vi "WraparoundUpdate.vi"(9 "Data":i32[](array[numeric]), 10 "Location":u32, 11 "Accumulator":i32[](array[numeric])) -> (2 "NewLocation":u32, 3 "Accumulated":i32[](array[numeric]))   [LabVIEW 2014]
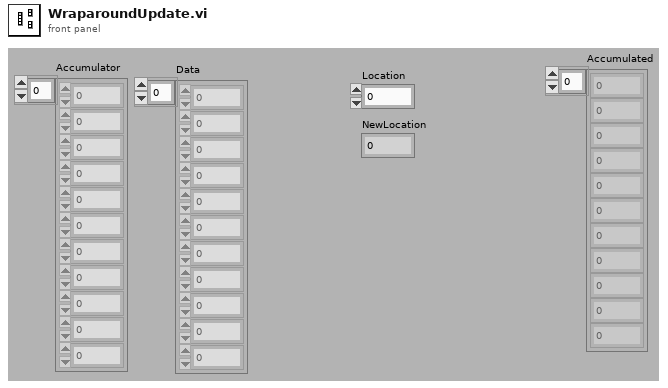
[diagram p1: front panel]
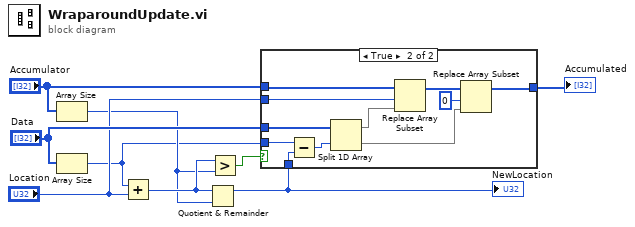
[diagram p0: block diagram]
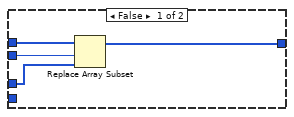
[diagram p2: hidden frame]
diagram:
  n1 = Array Size(array="Accumulator") -> (size(s)=w4:i32)
  n2 = Array Size(array="Data") -> (size(s)=w2:i32)
  n3 = Add(x=w2, y="Location") -> (x+y=w5:u32)
  n4 = Quotient & Remainder(x=w5, y=w4) -> (x-y*floor(x/y)=w1:u32)  [unwired: 1 out]
  "NewLocation" <- w1
  n5 = Greater?(x=w5, y=w4) -> (0:w3:bool)
  n6 = case shown="True" w3 {
    tunnel: "Data" -> [w12 w24]
    tunnel: "Accumulator" -> [w13 w20]
    tunnel: "Location" -> [w11 w19]
    tunnel: [w10 w14] -> w6
    tunnel: w2 -> [_ w23]
    tunnel: w1 -> [_ w22]
    frame False {
      n7 = Replace Array Subset(array=w13, new element=w12, index=w11) -> (w10:i32[])
    }
    frame True {
      n8 = Subtract(x=w23, y=w22) -> (x-y=w21:u32)
      n9 = Split 1D Array(array=w24, index=w21) -> (first subarray=w18:i32[], second subarray=w15:i32[])
      n10 = Replace Array Subset(array=w20, new element=w18, index=w19) -> (w17:i32[])
      n11 = Replace Array Subset(array=w17, new element=w15, index=0) -> (w14:i32[])
    }
  }
  "Accumulated" <- w6
